vi "Make Vis.vi"(11 "Map":T1) -> (3 "Vis":i32[][](array[numeric]))   [LabVIEW 2022 SP3, in "AoC22.lvlib"]
uses:
  AoC22.lvlib
  Map.ctl
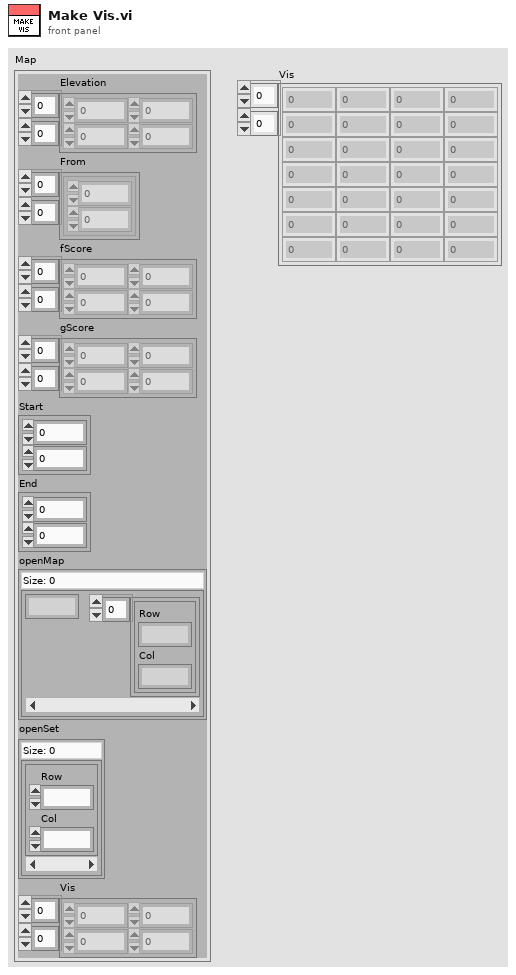
[diagram p1: front panel]
types:
  T1 = typedef "AoC22.lvlib/Map.ctl" = cluster{"Elevation":u8[][], "From":cluster{"Row":i32, "Col":i32}[][], "fScore":i32[][], "gScore":i32[][], "Start":cluster{"Row":i32, "Col":i32}, "End":cluster{"Row":i32, "Col":i32}, "openMap":map{i32, cluster{"Row":i32, "Col":i32}[]}, "openSet":set{cluster{"Row":i32, "Col":i32}}, "Vis":u8[][]}
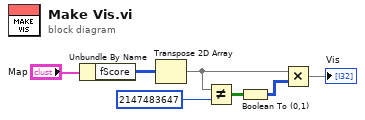
[diagram p0: block diagram]
diagram:
  n1 = Unbundle By Name("Map") -> ("fScore"=w7:i32[][])
  n2 = Transpose 2D Array(2D array=w7) -> (transposed array=w3:i32[][])
  n3 = Not Equal?(x=w3, y=2147483647) -> (x != y?=w4:bool[][])
  n4 = Boolean To (0,1)(Boolean=w4) -> (0, 1=w2:i16[][])
  n5 = Multiply(x=w3, y=w2) -> (x*y=→"Vis":i32[][])
